vi "DAQmx_Pulse_Countdown.vi"(8 "Number of Paired Pump-Probe Pulses":u32=500, 10 "CI.CountEdges.Term":tag="/Dev1/PFI0", 11 "counter":tag="Dev1/ctr0") -> ()   [LabVIEW 2025]
uses:
  <vilib>/DAQmx/read.llb/DAQmx Read (Counter U32 1Chan 1Samp).vi
  <vilib>/DAQmx/create/channels.llb/DAQmx Create Channel (CI-Count Edges).vi
  <vilib>/DAQmx/configure/timing.llb/DAQmx Timing (Sample Clock).vi
  <vilib>/DAQmx/miscellaneous.llb/DAQmx Fill In Error Info.vi
  <resource>/objmgr/daqmx.rc
  <vilib>/Utility/file.llb/Write Delimited Spreadsheet (DBL).vi
panel:
  out "Remaining Pulses":u32
  out "Array":dbl[](array[numeric]) format="%#_6f"
  out "Number of Counted Pulses":u32
  in  "CI.CountEdges.ActiveEdge":i32(ring)=10280 items=["Rising"=10280, "Falling"=10171]
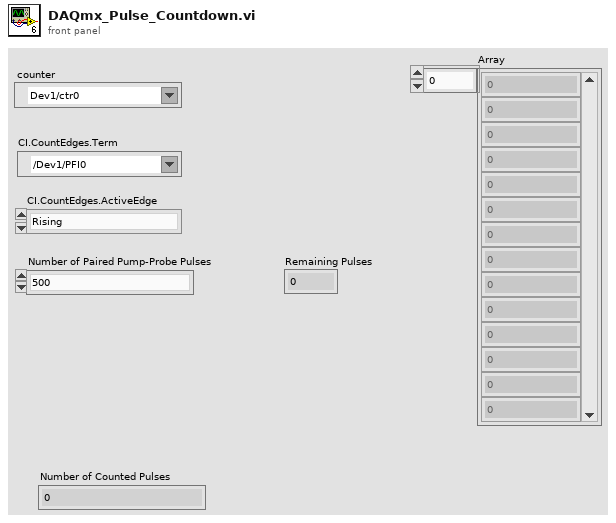
[diagram p1: front panel]
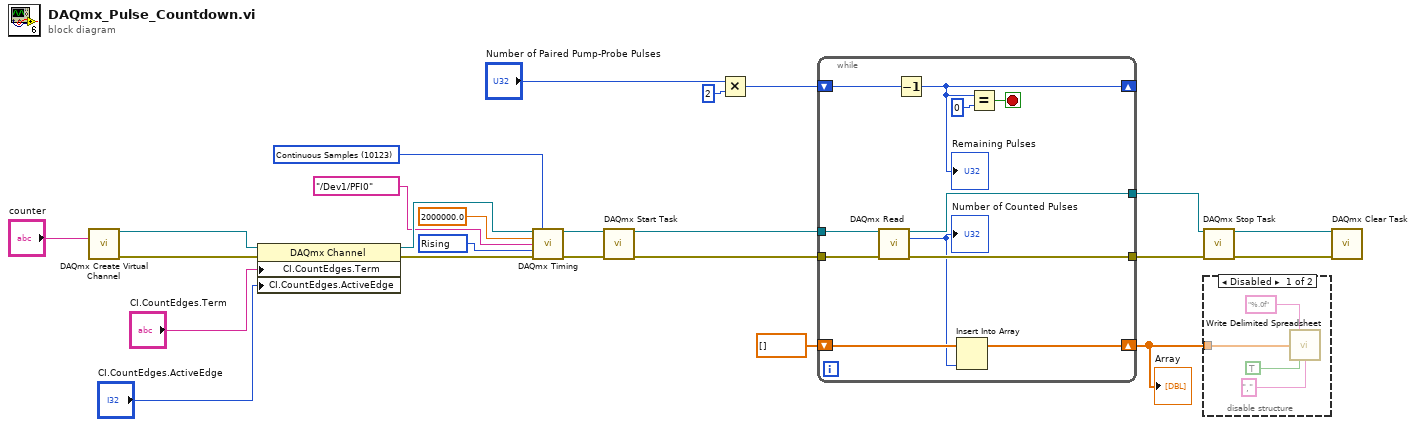
[diagram p0: block diagram]
diagram:
  w5 = 10280 items=["Rising"=10280, "Falling"=10171] ("active edge")
  w7 = 10123 items=["Finite Samples"=10178, "Continuous Samples"=10123, "Hardware Timed Single Point"=12522] ("sample mode")
  n1 = call-poly <vilib>:"DAQmx Create Virtual Channel.vi"("counter"="counter") -> ("task out"=w23:refnum<k21>, "error out"=w22:errorcluster)  [unwired: 13 in]
  n2 = property class="DAQmx Channel"(reference=w23, error in=w22, "CI.CountEdges.Term"="CI.CountEdges.Term", "CI.CountEdges.ActiveEdge"="CI.CountEdges.ActiveEdge") -> (reference out=w9:refnum<k21>, error out=w11:errorcluster)
  n3 = call-poly <vilib>:"DAQmx Timing.vi"("task/channels in"=w9, "sample mode"=w7, "rate"=2000000.0, "source"=tag "/Dev1/PFI0", "active edge"=w5, "error in"=w11) -> ("task out"=w8:refnum<k21>, "error out"=w10:errorcluster)  [unwired: 8 in]
  n4 = call <vilib>:"DAQmx Start Task.vi"("task/channels in"=w8, "error in"=w10) -> ("task out"=w20:refnum<k21>, "error out"=w19:errorcluster)  [unwired: 12 in]
  n5 = Multiply(x="Number of Paired Pump-Probe Pulses", y=u32 2) -> (x*y=w1:u32)
  n6 = while {
    tunnel: w20 -> [w34]
    tunnel: w19 -> [w33]
    tunnel: [w32] -> w18
    tunnel: [w31] -> w17
    shift-right: [w29] -> w12
    shift-left: dbl[] [] ("Array") -> [w30]
    shift-right: [w25] -> _
    shift-left: w1 -> [w26]
    stop <- w35 stop-if-true
    n7 = call-poly <vilib>:"DAQmx Read.vi"("task/channels in"=w34, "error in"=w33) -> ("task out"=w32:refnum<k21>, "data"=w28:u32, "error out"=w31:errorcluster)  [unwired: 11 in]
    "Number of Counted Pulses" <- w28
    n8 = Decrement(x=w26) -> (x-1=w25:u32)
    "Remaining Pulses" <- w25
    n9 = Insert Into Array(array=w30, new element=w28) -> (w29:dbl[])  [unwired: 1 in]
    n10 = Equal?(x=w25, y=u32 0) -> (x = y?=w35:bool)
  }
  "Array" <- w12
  n11 = call <vilib>:"DAQmx Stop Task.vi"("task/channels in"=w18, "error in"=w17) -> ("task out"=w16:refnum<k21>, "error out"=w15:errorcluster)  [unwired: 12 in]
  n12 = disable-structure shown="Disabled" {
    disable-tunnel: w12 -> [w39 _]
    frame Disabled {
      n13 = call-poly <vilib>:"Write Delimited Spreadsheet.vi"("format (%.3f)"="%.0f", "1D data"=w39, "transpose? (no:F)"=TRUE, "delimiter (\\t)"="," ("delimiter (\\t)")) -> ()  [unwired: 10 in, 2 out]
    }
    frame Enabled {
    }
  }
  n14 = call <vilib>:"DAQmx Clear Task.vi"("task in"=w16, "error in"=w15) -> ()  [unwired: 13 in, 1 out]
